vi "stop_sweep.vi"(8 "error in (no error)":errorcluster, 11 "DL090430TriggeredExperimentController in":refnum<class "ExperimentControllerDL090430DAQmxTriggered.lvclass">) -> (0 "error out":errorcluster, 3 "DL090430TriggeredExperimentController out":refnum<class "ExperimentControllerDL090430DAQmxTriggered.lvclass">)   [LabVIEW 2010, in "ExperimentControllerDL090430DAQmxTriggered.lvclass"]
uses:
  ExperimentControllerDL090430DAQmxTriggered.lvclass
  ImagingMode/GenericImagingMode/GenericImagingMode/GenericImagingMode.lvclass
  DataCollection/GenericDataCollection/GenericDataCollection/GenericDataCollection.lvclass
  DataCollection/GenericDataCollection/GenericDataCollection/trigger_enum.ctl
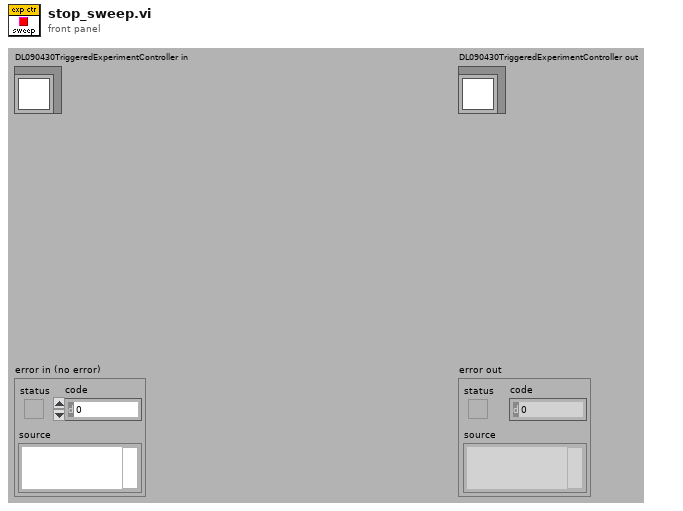
[diagram p1: front panel]
types:
  T1 = typedef "GenericDataCollection.lvclass/trigger_enum.ctl" = enum16{"NULL", "save", "reset"}
  T2 = typedef "GenericToplevelComponent.lvclass/common_trigger_enum.ctl" = enum16{"NULL", "initialise", "terminate", "fetch command", "fetch data", "attach observer", "register as observer", "detach observer", "acknowledge", "start", "stop", "sweep started", "sweep finished", "experiment started", "experiment stopped"}
  T3 = typedef "ExperimentControllerDL090430DAQmxTriggered.lvclass/mode_enum.ctl" = enum16{"trigger", "gate"}
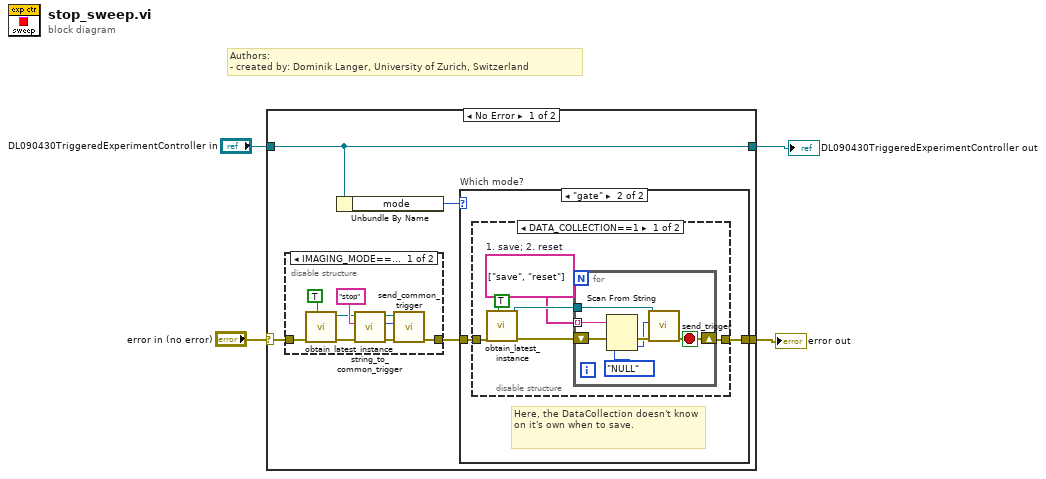
[diagram p0: block diagram]
diagram:
  # "Authors: \n- created by: Dominik Langer, University of Zurich, Switzerland"
  n1 = case shown="No Error" "error in (no error)" {
    selector: "error in (no error)" -> [w9 w38]
    tunnel: [w7 w38] -> w3
    tunnel: [w6 w37] -> w1
    tunnel: "DL090430TriggeredExperimentController in" -> [w6 w37]
    frame No Error {
      n2 = disable-structure shown="IMAGING_MODE==1" {
        disable-tunnel: w9 -> [w35 w36]
        disable-tunnel: [w34 w36] -> w8
        frame condition #0 (active) {
          n3 = call "obtain_latest_instance.vi"("quick, but maybe outdated?"=TRUE, "error in (no error)"=w35) -> ("error out"=w31:errorcluster, "GenericScanMode out"=w29:refnum<class "GenericImagingMode.lvclass">)  [unwired: 8 in]
          n4 = call-dynamic "string_to_common_trigger.vi"("error in (no error)"=w31, "trigger string"="stop", "GenericToplevelComponent in"=w29) -> ("error out"=w30:errorcluster, "trigger"=w27:T2, "GenericToplevelComponent out"=w28:refnum<class "GenericImagingMode.lvclass">)  [unwired: 6 in]
          n5 = call-dynamic "send_common_trigger.vi"("error in (no error)"=w30, "trigger"=w27, "GenericToplevelComponent in"=w28) -> ("error out"=w34:errorcluster)  [unwired: 6 in, 2 out]
        }
        frame condition #1 {
        }
      }
      n6 = Unbundle By Name(w6) -> ("mode"=w5:T3)
      n7 = case "Which mode?" shown="\"gate\"" w5 {
        tunnel: w8 -> [w10 w12]
        tunnel: [w10 w11] -> w7
        frame "trigger", Default {
        }
        frame "gate" {
          # "Here, the DataCollection doesn't know on it's own when to save."
          n8 = disable-structure shown="DATA_COLLECTION==1" {
            disable-tunnel: [w17 w26] -> w11
            disable-tunnel: w12 -> [w18 w26]
            frame condition #0 (active) {
              w14 = string[] ["save", "reset"]  # 1. save; 2. reset
              n9 = call "obtain_latest_instance.vi"("quick, but maybe outdated?"=TRUE, "error in (no error)"=w18) -> ("error out"=w16:errorcluster, "GenericDataCollection out"=w15:refnum<class "GenericDataCollection.lvclass">)  [unwired: 8 in]
              n10 = for {
                tunnel: w14 -> [w22] mode=indexing
                tunnel: w15 -> [w21]
                shift-right: [w25] -> w17
                shift-left: w16 -> [w24]
                stop <- w25 stop-if-true
                n11 = Scan From String(input string=w22, error in=w24, default 1=trigger_enum."NULL" ("trigger")) -> (error out=w23:errorcluster, output 1=w19:T1)  [unwired: 2 in, 2 out]
                n12 = call-dynamic "send_trigger.vi"("error in (no error)"=w23, "trigger"=w19, "GenericDataCollection in"=w21) -> ("error out"=w25:errorcluster)  [unwired: 7 in, 1 out]
              }
            }
            frame condition #1 {
            }
          }
        }
      }
    }
    frame Error {
    }
  }
  "error out" <- w3
  "DL090430TriggeredExperimentController out" <- w1
